vi "Read Data folder pathname.vi"() -> (0 "Data folder pathname.":path, 1 "PASS/FAIL.":bool)   [LabVIEW 2010]
panel:
  # "No inputs:"
  # "Outputs."
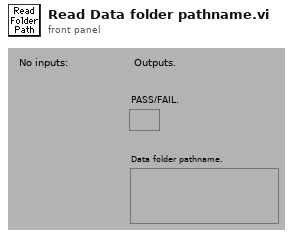
[diagram p1: front panel]
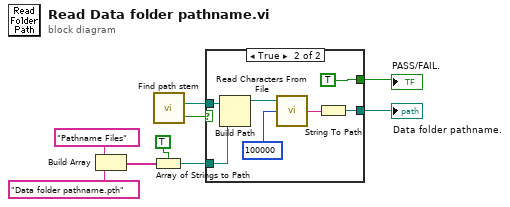
[diagram p0: block diagram]
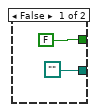
[diagram p2: hidden frame]
diagram:
  n1 = Build Array("Pathname Files", "Data folder pathname.pth") -> (w6:string[])
  n2 = Array of Strings to Path(0:w6, 1:TRUE) -> (2:w9:path)
  n3 = call "Find path stem.vi"() -> ("PASS/FAIL"=w8:bool, "Path stem."=w7:path)
  n4 = case shown="True" w8 {
    tunnel: w7 -> [_ w18]
    tunnel: w9 -> [_ w17]
    tunnel: [FALSE TRUE] -> w2
    tunnel: [path "" w12] -> w1
    frame False {
    }
    frame True {
      n5 = Build Path(base path=w18, name or relative path=w17) -> (appended path=w15:path)
      n6 = call <vilib>:"Read Characters From File.vi"("file path (dialog if empty)"=w15, "number of characters (all:-1)"=100000) -> ("character string"=w13:string)  [unwired: 7 out]
      n7 = String To Path(string=w13) -> (path=w12:path)
    }
  }
  "Data folder pathname." <- w1
  "PASS/FAIL." <- w2
